vi "Host.vi"() -> ()   [LabVIEW 2018]
uses:
  <instrlib>/niDCPower/nidcpower.llb/niDCPower Measurement Type.ctl
  <instrlib>/niScope/Configure/Trigger/niScope Configure Trigger Window.vi
  <instrlib>/niScope/Acquire/Fetch/niScope Multi Fetch Cluster.vi
  <instrlib>/niScope/Acquire/Fetch/niScope Fetch.vi
panel:
  in  "Tab Control":enum32{"Приборная панель", "Отладочная панель"}(tab)
  in  "STOP":bool=TRUE
  in  "Trigger Source":string(combo)="0"
  in  "AC/DC/Groun":i32(ring)=1 items=["AC", "DC", "Ground"]
  in  "Channel for SEU":T1(radio)
  in  "NI Scope":refnum<k15>="PXI1Slot5_2" caption="Scope"
  in  "High Level":dbl=0.2 format="%.2f"
  in  "Low Level":dbl=-0.2 format="%.2f"
  out "SEU_warning":bool caption="Find SEL"
  out "SEU_Counter":u32 caption="SEU counter"
  out "SEU Waveform":T2(graph) caption="SHUTDOWN Waveform"
  out "RealTime Waveform":T2(graph)=[{"relativeInitialX"=-0.00019999652392947102, "xIncrement"=4e-09, "wfm"=array[100000 elements]}] caption="PC_MON Waveform"
  out "P2 CH1_warning":bool caption="VCC_warning"
  out "P2 CH1_counter":u32 caption="VCC_counter"
  in  "P2 CH1_selcur, A":dbl=0.05 caption="current limit" format="%_6p"
  in  "P2 CH1 Used":bool
  in  "P2 CH1":bool
  out "P2 CH1_char":dbl(graph)=4.1881856349625015e-07
  in  "P2 CH1, V":dbl caption="voltage level" format="%_6p"
  out "P2 CH1_cur, A":dbl=4.1881856349625015e-07 caption="measurement" format="%_6g"
  in  "P2 CH1_curlim, A":dbl=0.1 caption="current limit" format="%_6p"
  out "SEL":bool
  in  "P1 CH0_selcur, A":dbl=0.05 caption="current limit" format="%_6p"
  in  "P1 CH1_selcur, A":dbl=0.05 caption="current limit" format="%_6p"
  in  "P2 CH0_selcur, A":dbl=0.05 caption="current limit" format="%_6p"
  out "P2 CH0_counter":u32 caption="VCC_counter"
  out "P2 CH0_warning":bool caption="VCC_warning"
  out "P1 CH1_counter":u32 caption="VCC_counter"
  out "P1 CH1_warning":bool caption="VCC_warning"
  out "P1 CH0_counter":u32 caption="VCC_counter"
  out "P1 CH0_warning":bool caption="VCC_warning"
  in  "SIM_SEL":bool
  in  "P2 CH0":bool
  in  "P1 CH1":bool
  in  "P1 CH0":bool
  in  "P2 CH0_curlim, A":dbl=0.1 caption="current limit" format="%_6p"
  out "P2 CH0_cur, A":dbl=8.408429577071082e-05 caption="measurement" format="%_6g"
  in  "P2 CH0, V":dbl caption="voltage level" format="%_6p"
  out "P2 CH0_char":dbl(graph)=8.408429577071082e-05
  in  "P1 CH1_curlim, A":dbl=0.1 caption="current limit" format="%_6p"
  out "P1CH1_cur, A":dbl=6.336785656464814e-07 caption="measurement" format="%_6g"
  in  "P1 CH1, V":dbl caption="voltage level" format="%_6p"
  out "P1 CH1_char":dbl(graph)=6.336785656464814e-07
  in  "P1 CH0_curlim, A":dbl=0.1 caption="current limit" format="%_6p"
  out "P1 CH0_cur, A":dbl=0.00010743246200593353 caption="measurement" format="%_6g"
  in  "P1 CH0, V":dbl caption="voltage level" format="%_6p"
  out "P1 CH0_char":dbl(graph)=8.030591065176734e-05
  out "Образец №":string
  in  "POWER 2 (CH0, CH1)":refnum<k15>="PXI1Slot3" caption="PRBS"
  in  "POWER 1 (CH0, CH1)":refnum<k15>="PXI1Slot2" caption="VСС_+5"
  in  "SEU":path=path "D:/NI LabVIEW/8939_VIL/SEU"
  in  "SEL":path=path "D:/NI LabVIEW/8939_VIL/SEL"
  in  "P1 CH0 Used":bool
  in  "P2 CH0 Used":bool
  in  "P1 CH1 Used":bool
  out "SEU last level":dbl
  out "SEU":bool caption="SEL"
  in  "SEL Time Cycle":u32=1
  out "Power OFF":bool
  in  "Считать SIM_SEL":bool
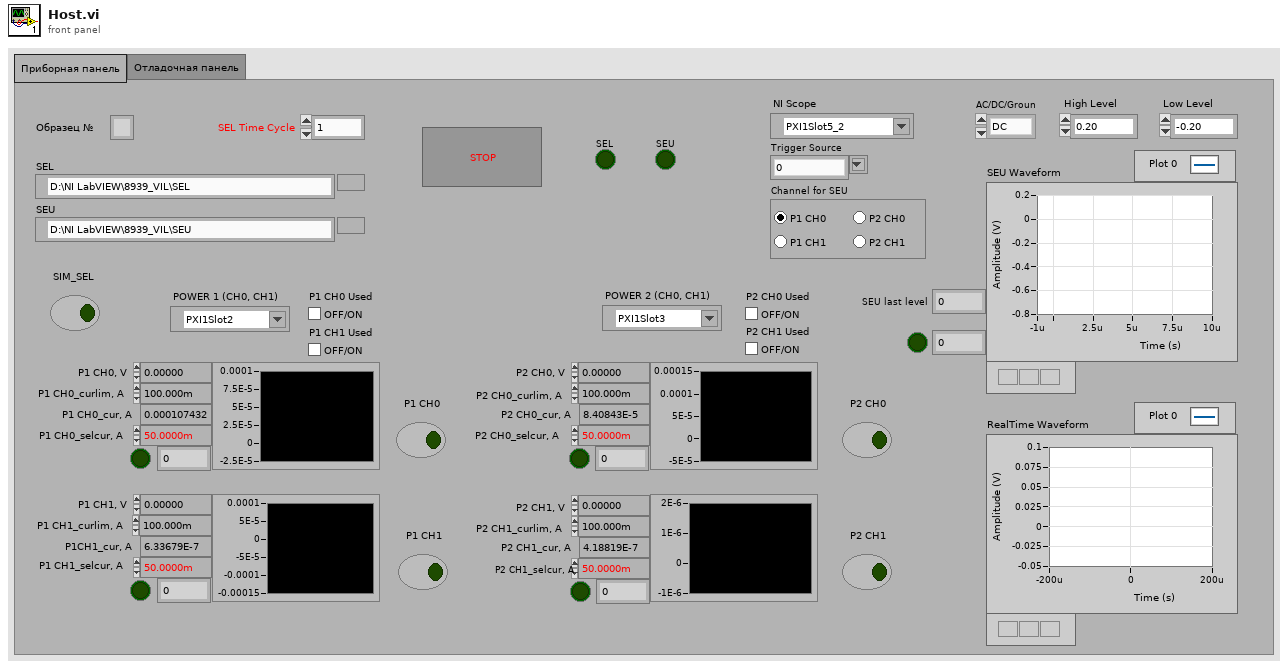
[diagram p1: front panel]
types:
  T1 = enum32{"Radio Selection P1 CH0", "Radio Selection P1 CH1", "Radio Selection P2 CH0", "Radio Selection P2 CH1"}
  T2 = cluster{"relativeInitialX":dbl, "xIncrement":dbl, "wfm":dbl[]}[]
  T3 = enum8{"Enabled", "Disabled", "Disabled and Grayed Out"}
  T4 = enum16{"open", "replace", "create", "open or create", "replace or create", "replace or create with confirmation"}
  T5 = typedef "niDCPower Measurement Type.ctl" = i32
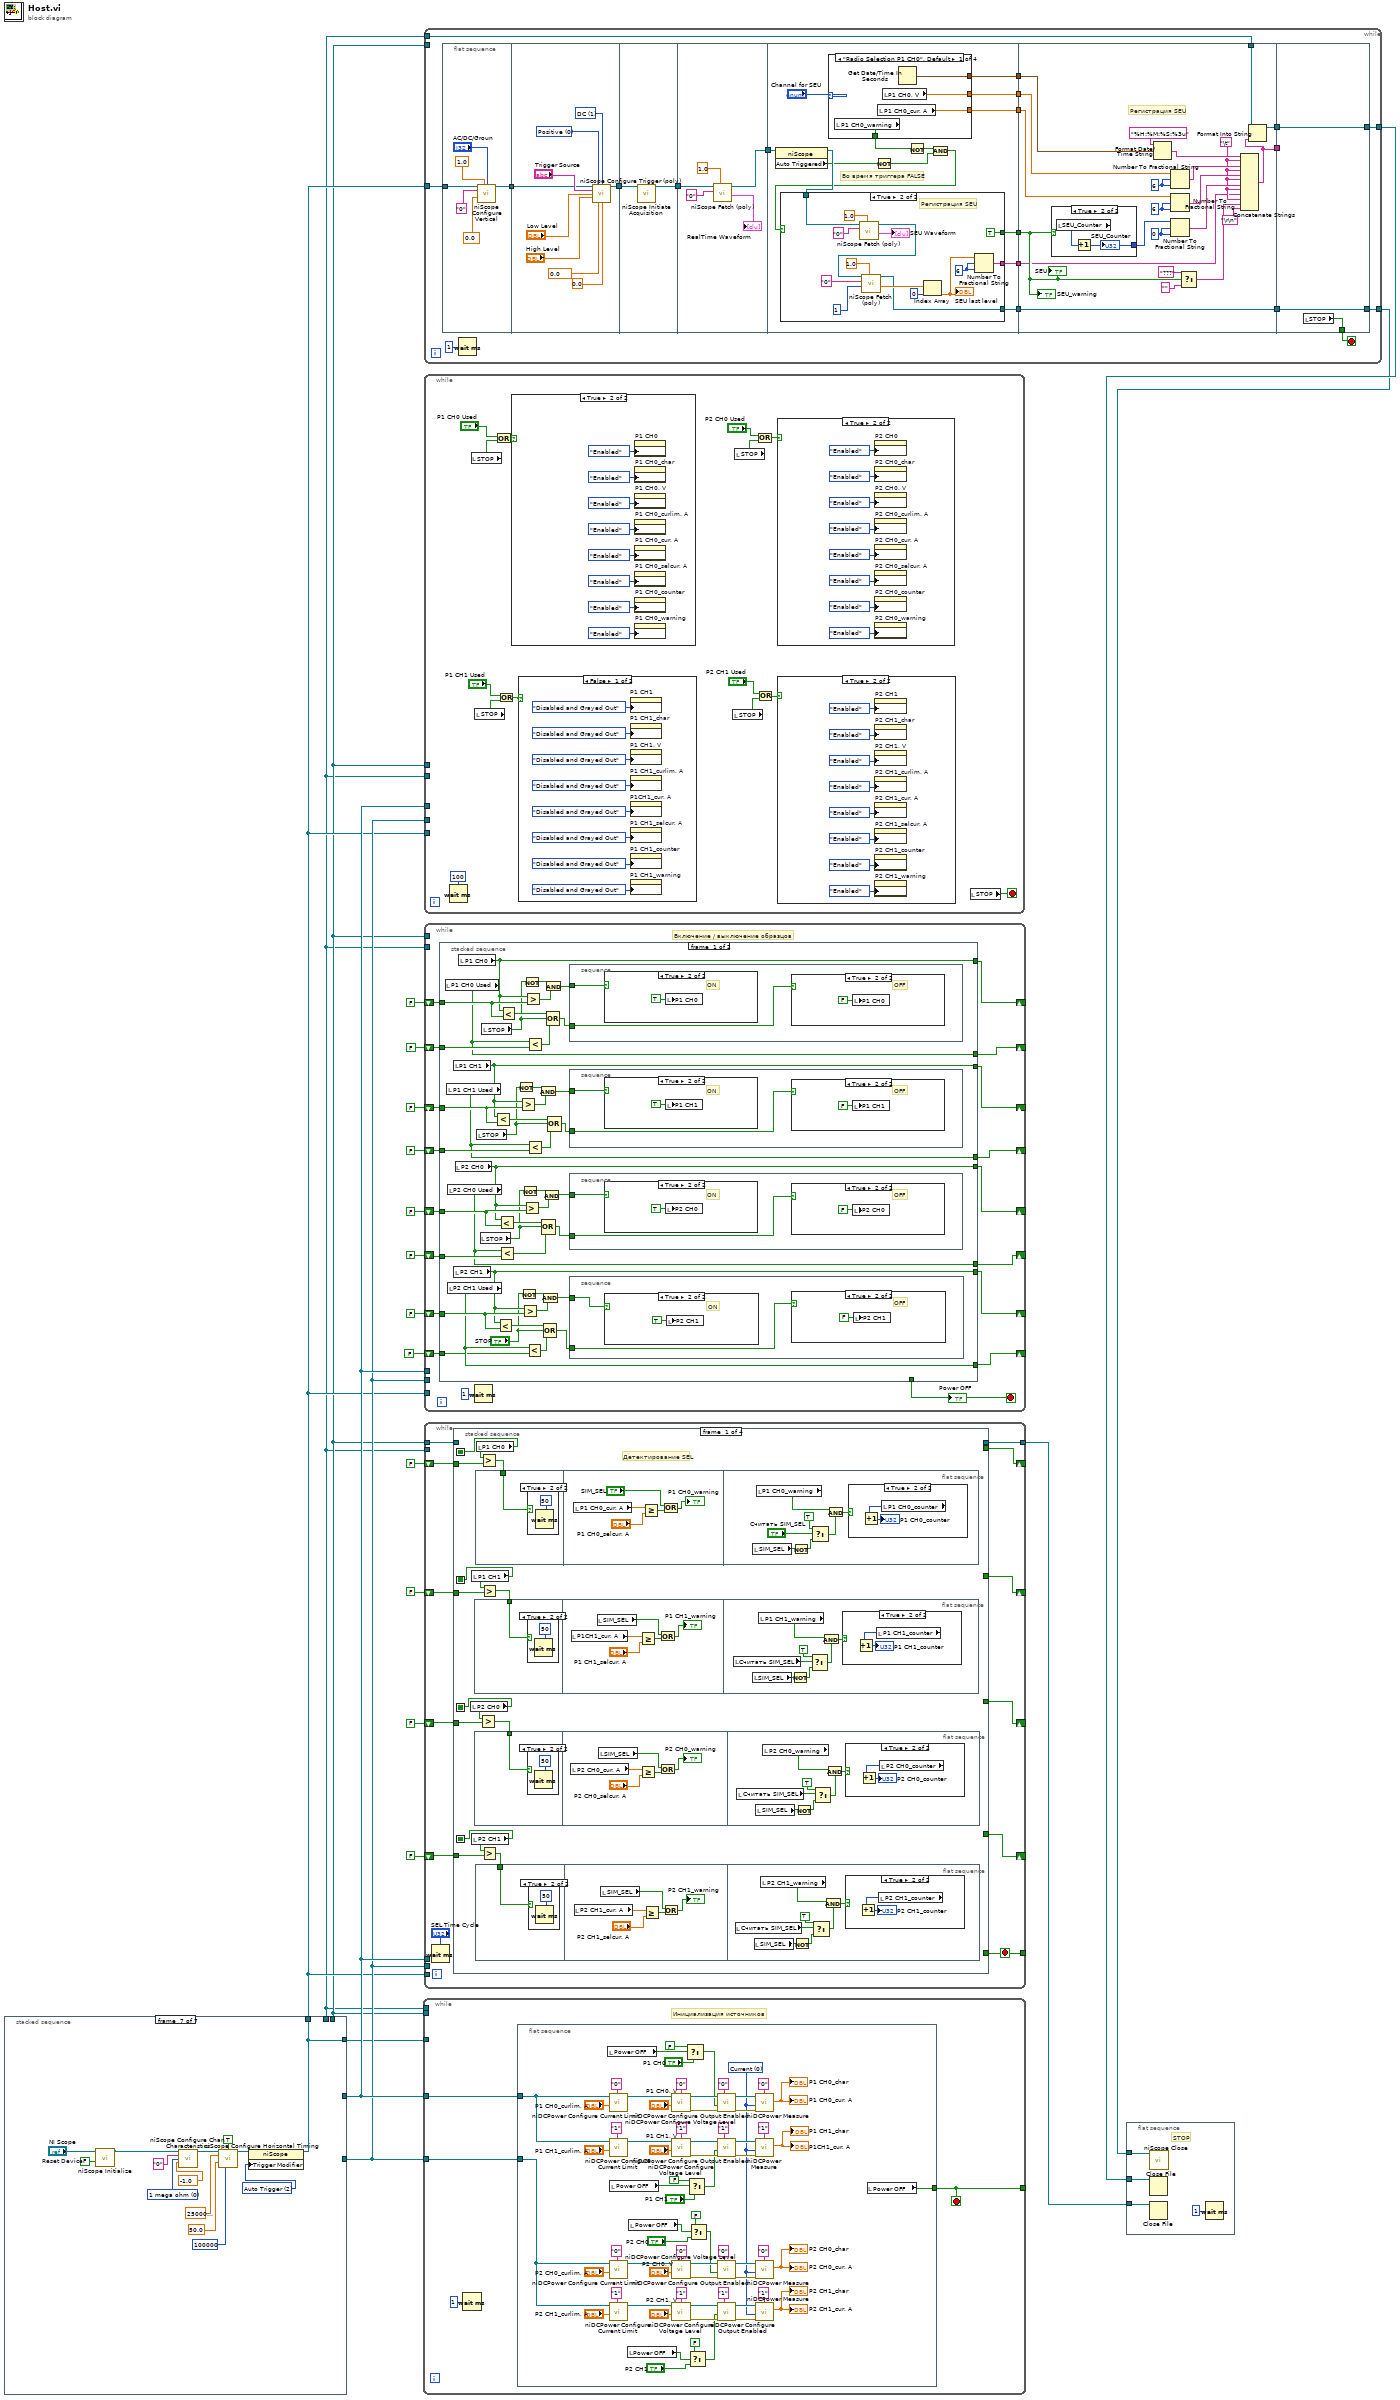
[diagram p0: block diagram]
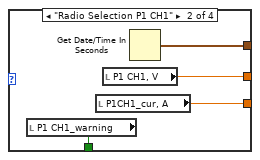
[diagram p2: hidden frame]
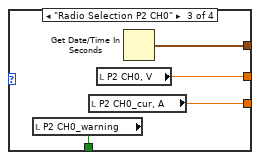
[diagram p3: hidden frame]
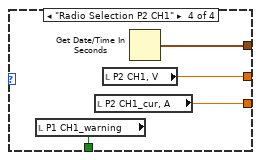
[diagram p4: hidden frame]
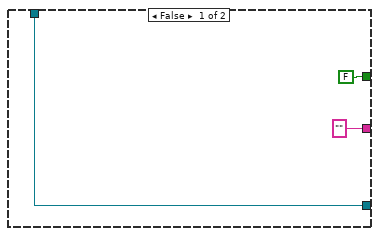
[diagram p5: hidden frame]
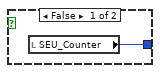
[diagram p6: hidden frame]
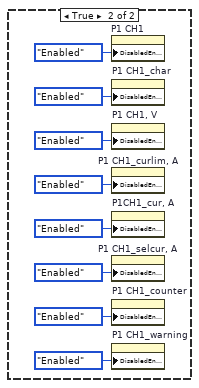
[diagram p7: hidden frame]
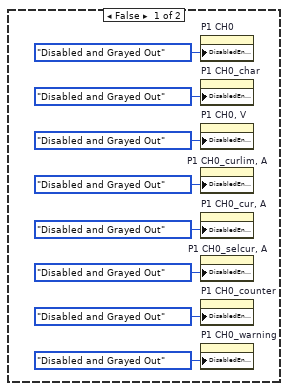
[diagram p8: hidden frame]
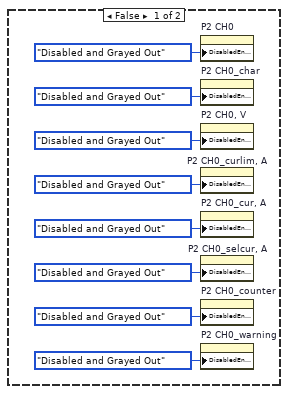
[diagram p9: hidden frame]
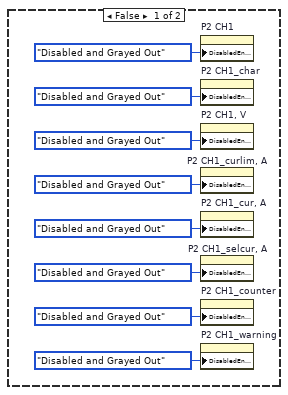
[diagram p10: hidden frame]
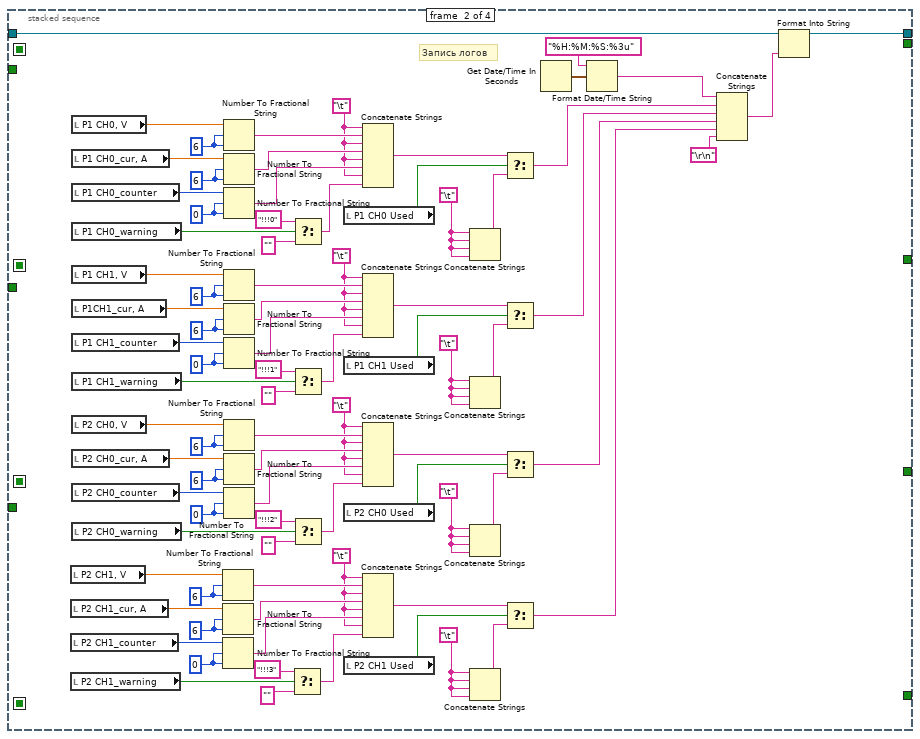
[diagram p19: hidden frame]
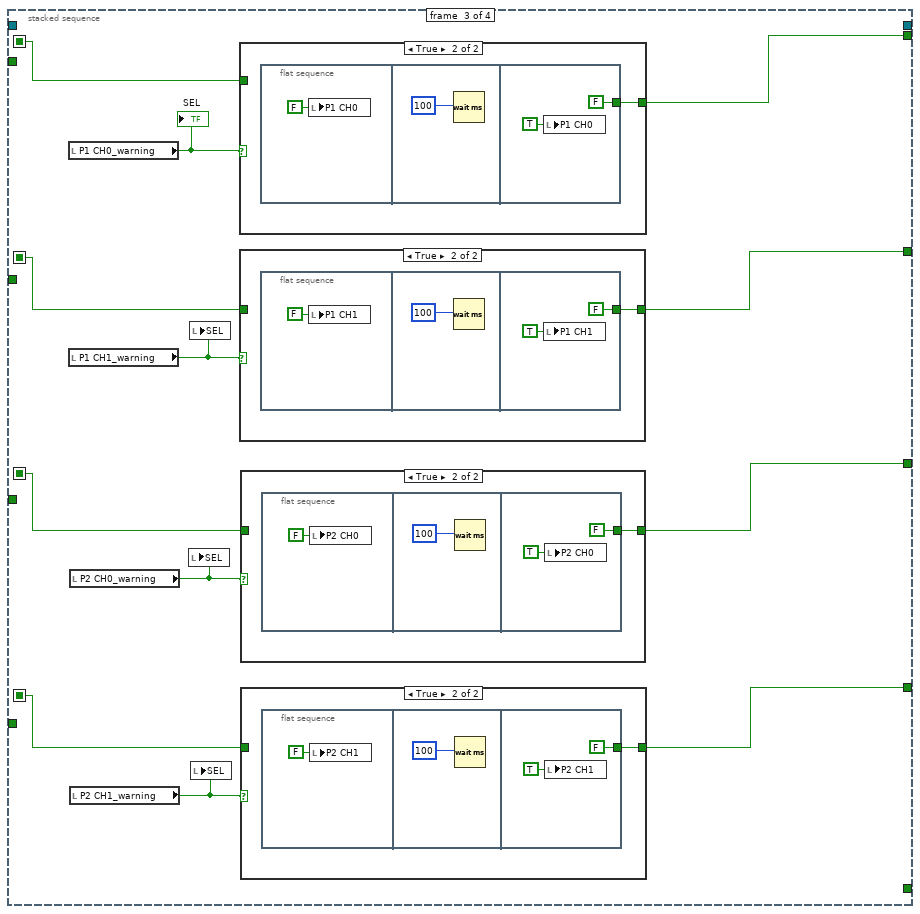
[diagram p20: hidden frame]
diagram:
  n1 = stacked-sequence {
    tunnel: [_ _ _ _ _ w164 _] -> w19
    tunnel: [_ _ _ _ _ w163 _] -> w18
    tunnel: [_ _ _ w97 _ _ _] -> w6
    tunnel: [_ _ _ _ _ _ w175] -> w11
    tunnel: [_ _ _ _ w138 _ _] -> w5
    tunnel: [_ _ _ _ _ _ w175] -> w10
    frame #0 {
      w23 = u32 0 ("SEU_Counter")
      w24 = FALSE ("STOP")
      # "Начальная конфигурация переменных"
      n2 = local write "STOP"(w24) -> ()
      n3 = local write "P1 CH0"(w24) -> ()
      n4 = local write "P1 CH1"(w24) -> ()
      n5 = local write "P2 CH0"(w24) -> ()
      n6 = local write "P2 CH1"(w24) -> ()
      n7 = local write "Power OFF"(w24) -> ()
      n8 = local write "P1 CH0 Used"(w24) -> ()
      n9 = local write "P1 CH1 Used"(w24) -> ()
      n10 = local write "P2 CH0 Used"(w24) -> ()
      n11 = local write "P2 CH1 Used"(w24) -> ()
      n12 = local write "Считать SIM_SEL"(w24) -> ()
      n13 = local write "SEL"(w24) -> ()
      n14 = local write "SEU"(w24) -> ()
      n15 = local write "SEU_warning"(w24) -> ()
      n16 = local write "P1 CH0_warning"(w24) -> ()
      n17 = local write "P1 CH1_warning"(w24) -> ()
      n18 = local write "P2 CH0_warning"(w24) -> ()
      n19 = local write "P2 CH1_warning"(w24) -> ()
      n20 = local write "SEU_warning"(w24) -> ()
      n21 = local write "SEU last level"(0.0 ("SEU Level")) -> ()
      n22 = local write "SEU_Counter"(w23) -> ()
      n23 = local write "P1 CH0_counter"(w23) -> ()
      n24 = local write "P1 CH1_counter"(w23) -> ()
      n25 = local write "P2 CH0_counter"(w23) -> ()
      n26 = local write "P2 CH1_counter"(w23) -> ()
      n27 = local write "Образец №"("" ("Образец №")) -> ()
    }
    frame #1 {
      n28 = stacked-sequence {
        frame #0 {
          n29 = local read "P1 CH0 Used"() -> (w26:bool)
          n30 = case shown="False" w26 {
            frame False {
              n31 = property on="P1 CH0" class="Bool (strict)"("DisabledEnum"=T3."Disabled and Grayed Out" ("Disabled")) -> ()  [unwired: 2 in, 2 out]
              n32 = property on="P1 CH0_char" class="WFChart (strict)"("DisabledEnum"=T3."Disabled and Grayed Out" ("Disabled")) -> ()  [unwired: 2 in, 2 out]
              n33 = property on="P1 CH0, V" class="DigNum (strict)"("DisabledEnum"=T3."Disabled and Grayed Out" ("Disabled")) -> ()  [unwired: 2 in, 2 out]
              n34 = property on="P1 CH0_curlim, A" class="DigNum (strict)"("DisabledEnum"=T3."Disabled and Grayed Out" ("Disabled")) -> ()  [unwired: 2 in, 2 out]
              n35 = property on="P1 CH0_cur, A" class="DigNum (strict)"("DisabledEnum"=T3."Disabled and Grayed Out" ("Disabled")) -> ()  [unwired: 2 in, 2 out]
              n36 = property on="P1 CH0_selcur, A" class="DigNum (strict)"("DisabledEnum"=T3."Disabled and Grayed Out" ("Disabled")) -> ()  [unwired: 2 in, 2 out]
              n37 = property on="P1 CH0_counter" class="DigNum (strict)"("DisabledEnum"=T3."Disabled and Grayed Out" ("Disabled")) -> ()  [unwired: 2 in, 2 out]
              n38 = property on="P1 CH0_warning" class="Bool (strict)"("DisabledEnum"=T3."Disabled and Grayed Out" ("Disabled")) -> ()  [unwired: 2 in, 2 out]
            }
            frame True {
              n39 = property on="P1 CH0" class="Bool (strict)"("DisabledEnum"=T3."Enabled" ("Disabled")) -> ()  [unwired: 2 in, 2 out]
              n40 = property on="P1 CH0_char" class="WFChart (strict)"("DisabledEnum"=T3."Enabled" ("Disabled")) -> ()  [unwired: 2 in, 2 out]
              n41 = property on="P1 CH0, V" class="DigNum (strict)"("DisabledEnum"=T3."Enabled" ("Disabled")) -> ()  [unwired: 2 in, 2 out]
              n42 = property on="P1 CH0_curlim, A" class="DigNum (strict)"("DisabledEnum"=T3."Enabled" ("Disabled")) -> ()  [unwired: 2 in, 2 out]
              n43 = property on="P1 CH0_cur, A" class="DigNum (strict)"("DisabledEnum"=T3."Enabled" ("Disabled")) -> ()  [unwired: 2 in, 2 out]
              n44 = property on="P1 CH0_selcur, A" class="DigNum (strict)"("DisabledEnum"=T3."Enabled" ("Disabled")) -> ()  [unwired: 2 in, 2 out]
              n45 = property on="P1 CH0_counter" class="DigNum (strict)"("DisabledEnum"=T3."Enabled" ("Disabled")) -> ()  [unwired: 2 in, 2 out]
              n46 = property on="P1 CH0_warning" class="Bool (strict)"("DisabledEnum"=T3."Enabled" ("Disabled")) -> ()  [unwired: 2 in, 2 out]
            }
          }
        }
        frame #1 {
          n47 = local read "P1 CH1 Used"() -> (w43:bool)
          n48 = case shown="False" w43 {
            frame False {
              n49 = property on="P1 CH1" class="Bool (strict)"("DisabledEnum"=T3."Disabled and Grayed Out" ("Disabled")) -> ()  [unwired: 2 in, 2 out]
              n50 = property on="P1 CH1_char" class="WFChart (strict)"("DisabledEnum"=T3."Disabled and Grayed Out" ("Disabled")) -> ()  [unwired: 2 in, 2 out]
              n51 = property on="P1 CH1, V" class="DigNum (strict)"("DisabledEnum"=T3."Disabled and Grayed Out" ("Disabled")) -> ()  [unwired: 2 in, 2 out]
              n52 = property on="P1 CH1_curlim, A" class="DigNum (strict)"("DisabledEnum"=T3."Disabled and Grayed Out" ("Disabled")) -> ()  [unwired: 2 in, 2 out]
              n53 = property on="P1CH1_cur, A" class="DigNum (strict)"("DisabledEnum"=T3."Disabled and Grayed Out" ("Disabled")) -> ()  [unwired: 2 in, 2 out]
              n54 = property on="P1 CH1_selcur, A" class="DigNum (strict)"("DisabledEnum"=T3."Disabled and Grayed Out" ("Disabled")) -> ()  [unwired: 2 in, 2 out]
              n55 = property on="P1 CH1_counter" class="DigNum (strict)"("DisabledEnum"=T3."Disabled and Grayed Out" ("Disabled")) -> ()  [unwired: 2 in, 2 out]
              n56 = property on="P1 CH1_warning" class="Bool (strict)"("DisabledEnum"=T3."Disabled and Grayed Out" ("Disabled")) -> ()  [unwired: 2 in, 2 out]
            }
            frame True {
              n57 = property on="P1 CH1" class="Bool (strict)"("DisabledEnum"=T3."Enabled" ("Disabled")) -> ()  [unwired: 2 in, 2 out]
              n58 = property on="P1 CH1_char" class="WFChart (strict)"("DisabledEnum"=T3."Enabled" ("Disabled")) -> ()  [unwired: 2 in, 2 out]
              n59 = property on="P1 CH1, V" class="DigNum (strict)"("DisabledEnum"=T3."Enabled" ("Disabled")) -> ()  [unwired: 2 in, 2 out]
              n60 = property on="P1 CH1_curlim, A" class="DigNum (strict)"("DisabledEnum"=T3."Enabled" ("Disabled")) -> ()  [unwired: 2 in, 2 out]
              n61 = property on="P1CH1_cur, A" class="DigNum (strict)"("DisabledEnum"=T3."Enabled" ("Disabled")) -> ()  [unwired: 2 in, 2 out]
              n62 = property on="P1 CH1_selcur, A" class="DigNum (strict)"("DisabledEnum"=T3."Enabled" ("Disabled")) -> ()  [unwired: 2 in, 2 out]
              n63 = property on="P1 CH1_counter" class="DigNum (strict)"("DisabledEnum"=T3."Enabled" ("Disabled")) -> ()  [unwired: 2 in, 2 out]
              n64 = property on="P1 CH1_warning" class="Bool (strict)"("DisabledEnum"=T3."Enabled" ("Disabled")) -> ()  [unwired: 2 in, 2 out]
            }
          }
        }
        frame #2 {
          n65 = local read "P2 CH0 Used"() -> (w60:bool)
          n66 = case shown="False" w60 {
            frame False {
              n67 = property on="P2 CH0" class="Bool (strict)"("DisabledEnum"=T3."Disabled and Grayed Out" ("Disabled")) -> ()  [unwired: 2 in, 2 out]
              n68 = property on="P2 CH0_char" class="WFChart (strict)"("DisabledEnum"=T3."Disabled and Grayed Out" ("Disabled")) -> ()  [unwired: 2 in, 2 out]
              n69 = property on="P2 CH0, V" class="DigNum (strict)"("DisabledEnum"=T3."Disabled and Grayed Out" ("Disabled")) -> ()  [unwired: 2 in, 2 out]
              n70 = property on="P2 CH0_curlim, A" class="DigNum (strict)"("DisabledEnum"=T3."Disabled and Grayed Out" ("Disabled")) -> ()  [unwired: 2 in, 2 out]
              n71 = property on="P2 CH0_cur, A" class="DigNum (strict)"("DisabledEnum"=T3."Disabled and Grayed Out" ("Disabled")) -> ()  [unwired: 2 in, 2 out]
              n72 = property on="P2 CH0_selcur, A" class="DigNum (strict)"("DisabledEnum"=T3."Disabled and Grayed Out" ("Disabled")) -> ()  [unwired: 2 in, 2 out]
              n73 = property on="P2 CH0_counter" class="DigNum (strict)"("DisabledEnum"=T3."Disabled and Grayed Out" ("Disabled")) -> ()  [unwired: 2 in, 2 out]
              n74 = property on="P2 CH0_warning" class="Bool (strict)"("DisabledEnum"=T3."Disabled and Grayed Out" ("Disabled")) -> ()  [unwired: 2 in, 2 out]
            }
            frame True {
              n75 = property on="P2 CH0" class="Bool (strict)"("DisabledEnum"=T3."Enabled" ("Disabled")) -> ()  [unwired: 2 in, 2 out]
              n76 = property on="P2 CH0_char" class="WFChart (strict)"("DisabledEnum"=T3."Enabled" ("Disabled")) -> ()  [unwired: 2 in, 2 out]
              n77 = property on="P2 CH0, V" class="DigNum (strict)"("DisabledEnum"=T3."Enabled" ("Disabled")) -> ()  [unwired: 2 in, 2 out]
              n78 = property on="P2 CH0_curlim, A" class="DigNum (strict)"("DisabledEnum"=T3."Enabled" ("Disabled")) -> ()  [unwired: 2 in, 2 out]
              n79 = property on="P2 CH0_cur, A" class="DigNum (strict)"("DisabledEnum"=T3."Enabled" ("Disabled")) -> ()  [unwired: 2 in, 2 out]
              n80 = property on="P2 CH0_selcur, A" class="DigNum (strict)"("DisabledEnum"=T3."Enabled" ("Disabled")) -> ()  [unwired: 2 in, 2 out]
              n81 = property on="P2 CH0_counter" class="DigNum (strict)"("DisabledEnum"=T3."Enabled" ("Disabled")) -> ()  [unwired: 2 in, 2 out]
              n82 = property on="P2 CH0_warning" class="Bool (strict)"("DisabledEnum"=T3."Enabled" ("Disabled")) -> ()  [unwired: 2 in, 2 out]
            }
          }
        }
        frame #3 {
          n83 = local read "P2 CH1 Used"() -> (w77:bool)
          n84 = case shown="True" w77 {
            frame False {
              n85 = property on="P2 CH1" class="Bool (strict)"("DisabledEnum"=T3."Disabled and Grayed Out" ("Disabled")) -> ()  [unwired: 2 in, 2 out]
              n86 = property on="P2 CH1_char" class="WFChart (strict)"("DisabledEnum"=T3."Disabled and Grayed Out" ("Disabled")) -> ()  [unwired: 2 in, 2 out]
              n87 = property on="P2 CH1, V" class="DigNum (strict)"("DisabledEnum"=T3."Disabled and Grayed Out" ("Disabled")) -> ()  [unwired: 2 in, 2 out]
              n88 = property on="P2 CH1_curlim, A" class="DigNum (strict)"("DisabledEnum"=T3."Disabled and Grayed Out" ("Disabled")) -> ()  [unwired: 2 in, 2 out]
              n89 = property on="P2 CH1_cur, A" class="DigNum (strict)"("DisabledEnum"=T3."Disabled and Grayed Out" ("Disabled")) -> ()  [unwired: 2 in, 2 out]
              n90 = property on="P2 CH1_selcur, A" class="DigNum (strict)"("DisabledEnum"=T3."Disabled and Grayed Out" ("Disabled")) -> ()  [unwired: 2 in, 2 out]
              n91 = property on="P2 CH1_counter" class="DigNum (strict)"("DisabledEnum"=T3."Disabled and Grayed Out" ("Disabled")) -> ()  [unwired: 2 in, 2 out]
              n92 = property on="P2 CH1_warning" class="Bool (strict)"("DisabledEnum"=T3."Disabled and Grayed Out" ("Disabled")) -> ()  [unwired: 2 in, 2 out]
            }
            frame True {
              n93 = property on="P2 CH1" class="Bool (strict)"("DisabledEnum"=T3."Enabled" ("Disabled")) -> ()  [unwired: 2 in, 2 out]
              n94 = property on="P2 CH1_char" class="WFChart (strict)"("DisabledEnum"=T3."Enabled" ("Disabled")) -> ()  [unwired: 2 in, 2 out]
              n95 = property on="P2 CH1, V" class="DigNum (strict)"("DisabledEnum"=T3."Enabled" ("Disabled")) -> ()  [unwired: 2 in, 2 out]
              n96 = property on="P2 CH1_curlim, A" class="DigNum (strict)"("DisabledEnum"=T3."Enabled" ("Disabled")) -> ()  [unwired: 2 in, 2 out]
              n97 = property on="P2 CH1_cur, A" class="DigNum (strict)"("DisabledEnum"=T3."Enabled" ("Disabled")) -> ()  [unwired: 2 in, 2 out]
              n98 = property on="P2 CH1_selcur, A" class="DigNum (strict)"("DisabledEnum"=T3."Enabled" ("Disabled")) -> ()  [unwired: 2 in, 2 out]
              n99 = property on="P2 CH1_counter" class="DigNum (strict)"("DisabledEnum"=T3."Enabled" ("Disabled")) -> ()  [unwired: 2 in, 2 out]
              n100 = property on="P2 CH1_warning" class="Bool (strict)"("DisabledEnum"=T3."Enabled" ("Disabled")) -> ()  [unwired: 2 in, 2 out]
            }
          }
        }
      }
    }
    frame #2 {
      n101 = call "Begin.vi"() -> ("Образец № 2"=→"Образец №":string)  [unwired: 9 in]
    }
    frame #3 {
      w96 = "\t"
      # "Инициализация файла SEL"
      n102 = local read "Образец №"() -> (w116:string)
      n103 = Build Path(base path="SEL", name or relative path=w116) -> (appended path=w131:path)
      n104 = Get Date/Time In Seconds() -> (seconds since 1Jan1904=w127:timestamp)
      n105 = call <vilib>:"Check if File or Folder Exists.vi"("path"=w131) -> ("file or folder exists?"=w130:bool, "dup path"=w129:path)  [unwired: 8 in, 1 out]
      n106 = Format Date/Time String(time format string (%c)="SEL %d %m %y %H.%M.%S", seconds (now)=w127) -> (date/time string=w126:string)  [unwired: 1 in]
      n107 = case shown="False" w130 {
        tunnel: w129 -> [w133 w134]
        tunnel: [w132 w134] -> w128
        frame False {
          n108 = Create Folder(path (use dialog)=w133) -> (created path=w132:path)  [unwired: 2 in, 2 out]
        }
        frame True {
        }
      }
      n109 = Concatenate Strings(w126, ".xls" ("string")) -> (w123:string)
      n110 = Build Path(base path=w128, name or relative path=w123) -> (appended path=w120:path)
      n111 = Open/Create/Replace File(file path (use dialog)=w120, operation (0:open)=T4."open or create", access (0:read/write)=enum16{"read/write", "read-only", "write-only"}."read/write") -> (refnum out=w119:refnum<file>)  [unwired: 3 in, 2 out]
      n112 = Set File Position(refnum=w119, from (0:start)=enum16{"start", "end", "current"}."end") -> (refnum out=w98:refnum<file>)  [unwired: 2 in, 1 out]
      n113 = Format Into String(initial string=w98, "Time" ("string"), w96, "P1 CH0, V" ("string"), w96, "P1 CH0_cur, A" ("string"), w96, "P1 CH0_counter" ("string"), w96, "!!!0" ("input 7"), w96, "P1 CH1, V" ("string"), w96, "P1 CH1_cur, A" ("string"), w96, "P1 CH1_counter" ("string"), w96, "!!!1" ("input 7"), w96, "P2 CH0, V" ("string"), w96, "P2 CH0_cur, A" ("string"), w96, "P2 CH0_counter" ("string"), w96, "!!!2" ("input 7"), w96, "P2 CH1, V" ("string"), w96, "P2 CH1_cur, A" ("string"), w96, "P2 CH1_counter" ("string"), "!!!3" ("input 7"), "\r\n") -> (resulting string=w97:refnum<file>)  [unwired: 2 in, 1 out]
    }
    frame #4 {
      w137 = "\t"
      # "Инициализация файла SEU"
      n114 = local read "Образец №"() -> (w149:string)
      n115 = Build Path(base path="SEU", name or relative path=w149) -> (appended path=w159:path)
      n116 = Get Date/Time In Seconds() -> (seconds since 1Jan1904=w155:timestamp)
      n117 = call <vilib>:"Check if File or Folder Exists.vi"("path"=w159) -> ("file or folder exists?"=w158:bool, "dup path"=w157:path)  [unwired: 8 in, 1 out]
      n118 = Format Date/Time String(time format string (%c)="SEU %d %m %y %H.%M.%S", seconds (now)=w155) -> (date/time string=w154:string)  [unwired: 1 in]
      n119 = case shown="False" w158 {
        tunnel: w157 -> [w161 w162]
        tunnel: [w160 w162] -> w156
        frame False {
          n120 = Create Folder(path (use dialog)=w161) -> (created path=w160:path)  [unwired: 2 in, 2 out]
        }
        frame True {
        }
      }
      n121 = Concatenate Strings(w154, ".xls" ("string")) -> (w153:string)
      n122 = Build Path(base path=w156, name or relative path=w153) -> (appended path=w152:path)
      n123 = Open/Create/Replace File(file path (use dialog)=w152, operation (0:open)=T4."open or create", access (0:read/write)=enum16{"read/write", "read-only", "write-only"}."read/write") -> (refnum out=w151:refnum<file>)  [unwired: 3 in, 2 out]
      n124 = Set File Position(refnum=w151, from (0:start)=enum16{"start", "end", "current"}."end") -> (refnum out=w139:refnum<file>)  [unwired: 2 in, 1 out]
      n125 = Format Into String(initial string=w139, "Time" ("string"), w137, "Voltage, V" ("string"), w137, "Current, A" ("string"), w137, "SEU counter" ("string"), w137, "!!!" ("input 7"), "\r\n") -> (resulting string=w138:refnum<file>)  [unwired: 2 in, 1 out]
    }
    frame #5 {
      # "Инициализация источника"
      n126 = call <instrlib>:"niDCPower Initialize.vi"("resource name"="POWER 1 (CH0, CH1)") -> ("error out"=w173:errorcluster, "instrument handle out"=w174:refnum<k15>)  [unwired: 3 in, 6 out]
      n127 = call <instrlib>:"niDCPower Initialize.vi"("resource name"="POWER 2 (CH0, CH1)") -> ("error out"=w170:errorcluster, "instrument handle out"=w171:refnum<k15>)  [unwired: 3 in, 6 out]
      n128 = call <instrlib>:"niDCPower Configure Voltage Level.vi"("error in (no error)"=w173, "voltage level"=0.0, "channel name"="0,1", "instrument handle"=w174) -> ("instrument handle out"=w164:refnum<k15>)  [unwired: 6 in, 1 out]
      n129 = call <instrlib>:"niDCPower Configure Voltage Level.vi"("error in (no error)"=w170, "voltage level"=0.0, "channel name"="0,1", "instrument handle"=w171) -> ("instrument handle out"=w163:refnum<k15>)  [unwired: 6 in, 1 out]
    }
    frame #6 {
      w179 = 2 items=["None"=1, "Auto Trigger"=2] ("Triggering:Trigger Modifier")
      w185 = u32 0 items=["1 mega ohm"=0, "50 ohms"=2] ("Input Impedance")
      w187 = FALSE  # Reset Device
      n130 = call <instrlib>:"niScope Initialize.vi"("resource name"="NI Scope", "reset device"=w187) -> ("instrument handle"=w176:refnum<k15>)  [unwired: 12 in, 1 out]
      n131 = call <instrlib>:"niScope Configure Chan Characteristics.vi"("instrument handle"=w176, "channels"="0" ("Channel Name"), "input impedance"=w185, "maximum input frequency"=-1.0 ("Maximum Input Frequency")) -> ("instrument handle out"=w178:refnum<k15>)  [unwired: 10 in, 1 out]
      n132 = call <instrlib>:"niScope Configure Horizontal Timing.vi"("instrument handle"=w178, "enforce realtime"=TRUE ("Enforce Realtime"), "min sample rate"=250000000.0 ("Min Sample Rate"), "reference position"=50.0 ("Reference\nPosition"), "min record length"=100000 ("Min Record Length")) -> ("instrument handle out"=w177:refnum<k15>)  [unwired: 9 in, 1 out]
      n133 = property on="Property Node" class="niScope"(reference=w177, "Trigger Modifier"=w179) -> (reference out=w175:refnum<k15>)  [unwired: 1 in, 1 out]
    }
  }
  n134 = while {
    tunnel: w19 -> [w192]
    tunnel: [w191] -> _
    tunnel: w18 -> [w189]
    tunnel: w10 -> [_]
    tunnel: w6 -> [_]
    tunnel: w5 -> [_]
    stop <- w191 stop-if-true
    # "Инициализация источников"
    n135 = Wait (ms)(milliseconds to wait=u32 1) -> ()  [unwired: 1 out]
    n136 = flat-sequence {
      tunnel: w192 -> [w260]
      tunnel: [w235] -> w191
      tunnel: w189 -> [w193]
      frame #0 {
        w194 = T5 0 items=["Current", "Voltage"] ("measurement type")
        n137 = local read "Power OFF"() -> (w212:bool)
        n138 = call <instrlib>:"niDCPower Configure Current Limit.vi"("current limit"="P1 CH0_curlim, A", "channel name"="0", "instrument handle"=w260) -> ("instrument handle out"=w249:refnum<k15>)  [unwired: 7 in, 1 out]
        n139 = call <instrlib>:"niDCPower Configure Current Limit.vi"("current limit"="P1 CH1_curlim, A", "channel name"="1", "instrument handle"=w260) -> ("instrument handle out"=w246:refnum<k15>)  [unwired: 7 in, 1 out]
        n140 = call <instrlib>:"niDCPower Configure Current Limit.vi"("current limit"="P2 CH0_curlim, A", "channel name"="0", "instrument handle"=w193) -> ("instrument handle out"=w225:refnum<k15>)  [unwired: 7 in, 1 out]
        n141 = call <instrlib>:"niDCPower Configure Current Limit.vi"("current limit"="P2 CH1_curlim, A", "channel name"="1", "instrument handle"=w193) -> ("instrument handle out"=w204:refnum<k15>)  [unwired: 7 in, 1 out]
        n142 = local read "Power OFF"() -> (w234:bool)
        n143 = local read "Power OFF"() -> (w197:bool)
        n144 = local read "Power OFF"() -> (w217:bool)
        n145 = call <instrlib>:"niDCPower Configure Voltage Level.vi"("voltage level"="P1 CH0, V", "channel name"="0", "instrument handle"=w249) -> ("error out"=w254:errorcluster, "instrument handle out"=w255:refnum<k15>)  [unwired: 7 in]
        n146 = call <instrlib>:"niDCPower Configure Voltage Level.vi"("voltage level"="P1 CH1, V", "channel name"="1", "instrument handle"=w246) -> ("error out"=w252:errorcluster, "instrument handle out"=w253:refnum<k15>)  [unwired: 7 in]
        n147 = call <instrlib>:"niDCPower Configure Voltage Level.vi"("voltage level"="P2 CH0, V", "channel name"="0", "instrument handle"=w225) -> ("error out"=w222:errorcluster, "instrument handle out"=w221:refnum<k15>)  [unwired: 7 in]
        n148 = call <instrlib>:"niDCPower Configure Voltage Level.vi"("voltage level"="P2 CH1, V", "channel name"="1", "instrument handle"=w204) -> ("error out"=w207:errorcluster, "instrument handle out"=w208:refnum<k15>)  [unwired: 7 in]
        n149 = Select(t=FALSE, s=w212, f="P1 CH0") -> (s? t:f=w211:bool)
        n150 = Select(t=FALSE, s=w234, f="P1 CH1") -> (s? t:f=w231:bool)
        n151 = Select(t=FALSE, s=w197, f="P2 CH1") -> (s? t:f=w195:bool)
        n152 = Select(t=FALSE, s=w217, f="P2 CH0") -> (s? t:f=w216:bool)
        n153 = call <instrlib>:"niDCPower Configure Output Enabled.vi"("error in (no error)"=w254, "output enabled"=w211, "channel name"="0", "instrument handle"=w255) -> ("error out"=w257:errorcluster, "instrument handle out"=w256:refnum<k15>)  [unwired: 6 in]
        n154 = call <instrlib>:"niDCPower Configure Output Enabled.vi"("error in (no error)"=w252, "output enabled"=w231, "channel name"="1", "instrument handle"=w253) -> ("error out"=w259:errorcluster, "instrument handle out"=w258:refnum<k15>)  [unwired: 6 in]
        n155 = call <instrlib>:"niDCPower Configure Output Enabled.vi"("error in (no error)"=w222, "output enabled"=w216, "channel name"="0", "instrument handle"=w221) -> ("error out"=w219:errorcluster, "instrument handle out"=w220:refnum<k15>)  [unwired: 6 in]
        n156 = call <instrlib>:"niDCPower Configure Output Enabled.vi"("error in (no error)"=w207, "output enabled"=w195, "channel name"="1", "instrument handle"=w208) -> ("error out"=w210:errorcluster, "instrument handle out"=w209:refnum<k15>)  [unwired: 6 in]
        n157 = call <instrlib>:"niDCPower Measure.vi"("error in (no error)"=w257, "measurement type"=w194, "channel name"="0", "instrument handle"=w256) -> ("measurement"=→"P1 CH0_cur, A" →"P1 CH0_char":dbl)  [unwired: 5 in, 2 out]
        n158 = call <instrlib>:"niDCPower Measure.vi"("error in (no error)"=w259, "measurement type"=w194, "channel name"="1", "instrument handle"=w258) -> ("measurement"=→"P1CH1_cur, A" →"P1 CH1_char":dbl)  [unwired: 5 in, 2 out]
        n159 = call <instrlib>:"niDCPower Measure.vi"("error in (no error)"=w219, "measurement type"=w194, "channel name"="0", "instrument handle"=w220) -> ("measurement"=→"P2 CH0_cur, A" →"P2 CH0_char":dbl)  [unwired: 5 in, 2 out]
        n160 = call <instrlib>:"niDCPower Measure.vi"("error in (no error)"=w210, "measurement type"=w194, "channel name"="1", "instrument handle"=w209) -> ("measurement"=→"P2 CH1_cur, A" →"P2 CH1_char":dbl)  [unwired: 5 in, 2 out]
        n161 = local read "Power OFF"() -> (w235:bool)
      }
    }
  }
  n162 = while {
    tunnel: w19 -> [_]
    tunnel: w18 -> [_]
    tunnel: w6 -> [_]
    tunnel: w5 -> [_]
    tunnel: w11 -> [_]
    stop <- w274 stop-if-true
    n163 = Wait (ms)(milliseconds to wait=u32 100) -> ()  [unwired: 1 out]
    n164 = local read "STOP"() -> (w264:bool)
    n165 = local read "STOP"() -> (w261:bool)
    n166 = Or(x="P1 CH0 Used", y=w264) -> (x .or. y?=w266:bool)
    n167 = Or(x="P1 CH1 Used", y=w261) -> (x .or. y?=w263:bool)
    n168 = case shown="True" w266 {
      frame False {
        n169 = property on="P1 CH0" class="Bool (strict)"("DisabledEnum"=T3."Disabled and Grayed Out" ("Disabled")) -> ()  [unwired: 2 in, 2 out]
        n170 = property on="P1 CH0_char" class="WFChart (strict)"("DisabledEnum"=T3."Disabled and Grayed Out" ("Disabled")) -> ()  [unwired: 2 in, 2 out]
        n171 = property on="P1 CH0, V" class="DigNum (strict)"("DisabledEnum"=T3."Disabled and Grayed Out" ("Disabled")) -> ()  [unwired: 2 in, 2 out]
        n172 = property on="P1 CH0_curlim, A" class="DigNum (strict)"("DisabledEnum"=T3."Disabled and Grayed Out" ("Disabled")) -> ()  [unwired: 2 in, 2 out]
        n173 = property on="P1 CH0_cur, A" class="DigNum (strict)"("DisabledEnum"=T3."Disabled and Grayed Out" ("Disabled")) -> ()  [unwired: 2 in, 2 out]
        n174 = property on="P1 CH0_selcur, A" class="DigNum (strict)"("DisabledEnum"=T3."Disabled and Grayed Out" ("Disabled")) -> ()  [unwired: 2 in, 2 out]
        n175 = property on="P1 CH0_counter" class="DigNum (strict)"("DisabledEnum"=T3."Disabled and Grayed Out" ("Disabled")) -> ()  [unwired: 2 in, 2 out]
        n176 = property on="P1 CH0_warning" class="Bool (strict)"("DisabledEnum"=T3."Disabled and Grayed Out" ("Disabled")) -> ()  [unwired: 2 in, 2 out]
      }
      frame True {
        n177 = property on="P1 CH0" class="Bool (strict)"("DisabledEnum"=T3."Enabled" ("Disabled")) -> ()  [unwired: 2 in, 2 out]
        n178 = property on="P1 CH0_char" class="WFChart (strict)"("DisabledEnum"=T3."Enabled" ("Disabled")) -> ()  [unwired: 2 in, 2 out]
        n179 = property on="P1 CH0, V" class="DigNum (strict)"("DisabledEnum"=T3."Enabled" ("Disabled")) -> ()  [unwired: 2 in, 2 out]
        n180 = property on="P1 CH0_curlim, A" class="DigNum (strict)"("DisabledEnum"=T3."Enabled" ("Disabled")) -> ()  [unwired: 2 in, 2 out]
        n181 = property on="P1 CH0_cur, A" class="DigNum (strict)"("DisabledEnum"=T3."Enabled" ("Disabled")) -> ()  [unwired: 2 in, 2 out]
        n182 = property on="P1 CH0_selcur, A" class="DigNum (strict)"("DisabledEnum"=T3."Enabled" ("Disabled")) -> ()  [unwired: 2 in, 2 out]
        n183 = property on="P1 CH0_counter" class="DigNum (strict)"("DisabledEnum"=T3."Enabled" ("Disabled")) -> ()  [unwired: 2 in, 2 out]
        n184 = property on="P1 CH0_warning" class="Bool (strict)"("DisabledEnum"=T3."Enabled" ("Disabled")) -> ()  [unwired: 2 in, 2 out]
      }
    }
    n185 = case shown="False" w263 {
      frame False {
        n186 = property on="P1 CH1" class="Bool (strict)"("DisabledEnum"=T3."Disabled and Grayed Out" ("Disabled")) -> ()  [unwired: 2 in, 2 out]
        n187 = property on="P1 CH1_char" class="WFChart (strict)"("DisabledEnum"=T3."Disabled and Grayed Out" ("Disabled")) -> ()  [unwired: 2 in, 2 out]
        n188 = property on="P1 CH1, V" class="DigNum (strict)"("DisabledEnum"=T3."Disabled and Grayed Out" ("Disabled")) -> ()  [unwired: 2 in, 2 out]
        n189 = property on="P1 CH1_curlim, A" class="DigNum (strict)"("DisabledEnum"=T3."Disabled and Grayed Out" ("Disabled")) -> ()  [unwired: 2 in, 2 out]
        n190 = property on="P1CH1_cur, A" class="DigNum (strict)"("DisabledEnum"=T3."Disabled and Grayed Out" ("Disabled")) -> ()  [unwired: 2 in, 2 out]
        n191 = property on="P1 CH1_selcur, A" class="DigNum (strict)"("DisabledEnum"=T3."Disabled and Grayed Out" ("Disabled")) -> ()  [unwired: 2 in, 2 out]
        n192 = property on="P1 CH1_counter" class="DigNum (strict)"("DisabledEnum"=T3."Disabled and Grayed Out" ("Disabled")) -> ()  [unwired: 2 in, 2 out]
        n193 = property on="P1 CH1_warning" class="Bool (strict)"("DisabledEnum"=T3."Disabled and Grayed Out" ("Disabled")) -> ()  [unwired: 2 in, 2 out]
      }
      frame True {
        n194 = property on="P1 CH1" class="Bool (strict)"("DisabledEnum"=T3."Enabled" ("Disabled")) -> ()  [unwired: 2 in, 2 out]
        n195 = property on="P1 CH1_char" class="WFChart (strict)"("DisabledEnum"=T3."Enabled" ("Disabled")) -> ()  [unwired: 2 in, 2 out]
        n196 = property on="P1 CH1, V" class="DigNum (strict)"("DisabledEnum"=T3."Enabled" ("Disabled")) -> ()  [unwired: 2 in, 2 out]
        n197 = property on="P1 CH1_curlim, A" class="DigNum (strict)"("DisabledEnum"=T3."Enabled" ("Disabled")) -> ()  [unwired: 2 in, 2 out]
        n198 = property on="P1CH1_cur, A" class="DigNum (strict)"("DisabledEnum"=T3."Enabled" ("Disabled")) -> ()  [unwired: 2 in, 2 out]
        n199 = property on="P1 CH1_selcur, A" class="DigNum (strict)"("DisabledEnum"=T3."Enabled" ("Disabled")) -> ()  [unwired: 2 in, 2 out]
        n200 = property on="P1 CH1_counter" class="DigNum (strict)"("DisabledEnum"=T3."Enabled" ("Disabled")) -> ()  [unwired: 2 in, 2 out]
        n201 = property on="P1 CH1_warning" class="Bool (strict)"("DisabledEnum"=T3."Enabled" ("Disabled")) -> ()  [unwired: 2 in, 2 out]
      }
    }
    n202 = local read "STOP"() -> (w270:bool)
    n203 = local read "STOP"() -> (w267:bool)
    n204 = Or(x="P2 CH0 Used", y=w267) -> (x .or. y?=w269:bool)
    n205 = Or(x="P2 CH1 Used", y=w270) -> (x .or. y?=w271:bool)
    n206 = case shown="True" w269 {
      frame False {
        n207 = property on="P2 CH0" class="Bool (strict)"("DisabledEnum"=T3."Disabled and Grayed Out" ("Disabled")) -> ()  [unwired: 2 in, 2 out]
        n208 = property on="P2 CH0_char" class="WFChart (strict)"("DisabledEnum"=T3."Disabled and Grayed Out" ("Disabled")) -> ()  [unwired: 2 in, 2 out]
        n209 = property on="P2 CH0, V" class="DigNum (strict)"("DisabledEnum"=T3."Disabled and Grayed Out" ("Disabled")) -> ()  [unwired: 2 in, 2 out]
        n210 = property on="P2 CH0_curlim, A" class="DigNum (strict)"("DisabledEnum"=T3."Disabled and Grayed Out" ("Disabled")) -> ()  [unwired: 2 in, 2 out]
        n211 = property on="P2 CH0_cur, A" class="DigNum (strict)"("DisabledEnum"=T3."Disabled and Grayed Out" ("Disabled")) -> ()  [unwired: 2 in, 2 out]
        n212 = property on="P2 CH0_selcur, A" class="DigNum (strict)"("DisabledEnum"=T3."Disabled and Grayed Out" ("Disabled")) -> ()  [unwired: 2 in, 2 out]
        n213 = property on="P2 CH0_counter" class="DigNum (strict)"("DisabledEnum"=T3."Disabled and Grayed Out" ("Disabled")) -> ()  [unwired: 2 in, 2 out]
        n214 = property on="P2 CH0_warning" class="Bool (strict)"("DisabledEnum"=T3."Disabled and Grayed Out" ("Disabled")) -> ()  [unwired: 2 in, 2 out]
      }
      frame True {
        n215 = property on="P2 CH0" class="Bool (strict)"("DisabledEnum"=T3."Enabled" ("Disabled")) -> ()  [unwired: 2 in, 2 out]
        n216 = property on="P2 CH0_char" class="WFChart (strict)"("DisabledEnum"=T3."Enabled" ("Disabled")) -> ()  [unwired: 2 in, 2 out]
        n217 = property on="P2 CH0, V" class="DigNum (strict)"("DisabledEnum"=T3."Enabled" ("Disabled")) -> ()  [unwired: 2 in, 2 out]
        n218 = property on="P2 CH0_curlim, A" class="DigNum (strict)"("DisabledEnum"=T3."Enabled" ("Disabled")) -> ()  [unwired: 2 in, 2 out]
        n219 = property on="P2 CH0_cur, A" class="DigNum (strict)"("DisabledEnum"=T3."Enabled" ("Disabled")) -> ()  [unwired: 2 in, 2 out]
        n220 = property on="P2 CH0_selcur, A" class="DigNum (strict)"("DisabledEnum"=T3."Enabled" ("Disabled")) -> ()  [unwired: 2 in, 2 out]
        n221 = property on="P2 CH0_counter" class="DigNum (strict)"("DisabledEnum"=T3."Enabled" ("Disabled")) -> ()  [unwired: 2 in, 2 out]
        n222 = property on="P2 CH0_warning" class="Bool (strict)"("DisabledEnum"=T3."Enabled" ("Disabled")) -> ()  [unwired: 2 in, 2 out]
      }
    }
    n223 = case shown="True" w271 {
      frame False {
        n224 = property on="P2 CH1" class="Bool (strict)"("DisabledEnum"=T3."Disabled and Grayed Out" ("Disabled")) -> ()  [unwired: 2 in, 2 out]
        n225 = property on="P2 CH1_char" class="WFChart (strict)"("DisabledEnum"=T3."Disabled and Grayed Out" ("Disabled")) -> ()  [unwired: 2 in, 2 out]
        n226 = property on="P2 CH1, V" class="DigNum (strict)"("DisabledEnum"=T3."Disabled and Grayed Out" ("Disabled")) -> ()  [unwired: 2 in, 2 out]
        n227 = property on="P2 CH1_curlim, A" class="DigNum (strict)"("DisabledEnum"=T3."Disabled and Grayed Out" ("Disabled")) -> ()  [unwired: 2 in, 2 out]
        n228 = property on="P2 CH1_cur, A" class="DigNum (strict)"("DisabledEnum"=T3."Disabled and Grayed Out" ("Disabled")) -> ()  [unwired: 2 in, 2 out]
        n229 = property on="P2 CH1_selcur, A" class="DigNum (strict)"("DisabledEnum"=T3."Disabled and Grayed Out" ("Disabled")) -> ()  [unwired: 2 in, 2 out]
        n230 = property on="P2 CH1_counter" class="DigNum (strict)"("DisabledEnum"=T3."Disabled and Grayed Out" ("Disabled")) -> ()  [unwired: 2 in, 2 out]
        n231 = property on="P2 CH1_warning" class="Bool (strict)"("DisabledEnum"=T3."Disabled and Grayed Out" ("Disabled")) -> ()  [unwired: 2 in, 2 out]
      }
      frame True {
        n232 = property on="P2 CH1" class="Bool (strict)"("DisabledEnum"=T3."Enabled" ("Disabled")) -> ()  [unwired: 2 in, 2 out]
        n233 = property on="P2 CH1_char" class="WFChart (strict)"("DisabledEnum"=T3."Enabled" ("Disabled")) -> ()  [unwired: 2 in, 2 out]
        n234 = property on="P2 CH1, V" class="DigNum (strict)"("DisabledEnum"=T3."Enabled" ("Disabled")) -> ()  [unwired: 2 in, 2 out]
        n235 = property on="P2 CH1_curlim, A" class="DigNum (strict)"("DisabledEnum"=T3."Enabled" ("Disabled")) -> ()  [unwired: 2 in, 2 out]
        n236 = property on="P2 CH1_cur, A" class="DigNum (strict)"("DisabledEnum"=T3."Enabled" ("Disabled")) -> ()  [unwired: 2 in, 2 out]
        n237 = property on="P2 CH1_selcur, A" class="DigNum (strict)"("DisabledEnum"=T3."Enabled" ("Disabled")) -> ()  [unwired: 2 in, 2 out]
        n238 = property on="P2 CH1_counter" class="DigNum (strict)"("DisabledEnum"=T3."Enabled" ("Disabled")) -> ()  [unwired: 2 in, 2 out]
        n239 = property on="P2 CH1_warning" class="Bool (strict)"("DisabledEnum"=T3."Enabled" ("Disabled")) -> ()  [unwired: 2 in, 2 out]
      }
    }
    n240 = local read "STOP"() -> (w274:bool)
  }
  n241 = while {
    shift-right: [w350] -> _
    shift-left: FALSE -> [w356]
    tunnel: w19 -> [_]
    tunnel: w18 -> [_]
    shift-right: [w349] -> _
    shift-left: FALSE -> [w355]
    shift-right: [w351] -> _
    shift-left: FALSE -> [w354]
    shift-right: [w352] -> _
    shift-left: FALSE -> [w353]
    tunnel: w6 -> [_]
    tunnel: w5 -> [_]
    tunnel: w11 -> [_]
    shift-right: [w345] -> _
    shift-left: FALSE -> [w346]
    shift-right: [w343] -> _
    shift-left: FALSE -> [w344]
    shift-right: [w341] -> _
    shift-left: FALSE -> [w342]
    shift-right: [w339] -> _
    shift-left: FALSE -> [w340]
    stop <- w347 stop-if-true
    # "Включение / выключение образцов"
    n242 = stacked-sequence {
      tunnel: w356 -> [w400 _]
      tunnel: [w396 _] -> w350
      tunnel: w355 -> [w392 _]
      tunnel: [w391 _] -> w349
      tunnel: w354 -> [w390 _]
      tunnel: w353 -> [w384 _]
      tunnel: [w382 _] -> w352
      tunnel: [w381 _] -> w351
      tunnel: [_ w417] -> w347
      tunnel: w346 -> [w378 _]
      tunnel: [w375 _] -> w345
      tunnel: w344 -> [w374 _]
      tunnel: [w369 _] -> w343
      tunnel: w342 -> [w364 _]
      tunnel: [w363 _] -> w341
      tunnel: w340 -> [w358 _]
      tunnel: [w359 _] -> w339
      frame #0 {
        n243 = local read "P1 CH0 Used"() -> (w375:bool)
        n244 = local read "P1 CH1 Used"() -> (w369:bool)
        n245 = local read "P2 CH0 Used"() -> (w363:bool)
        n246 = local read "P2 CH1 Used"() -> (w359:bool)
        n247 = local read "P1 CH1"() -> (w381:bool)
        n248 = local read "P2 CH1"() -> (w396:bool)
        n249 = local read "P2 CH0"() -> (w391:bool)
        n250 = local read "P1 CH0"() -> (w382:bool)
        n251 = local read "STOP"() -> (w371:bool)
        n252 = local read "STOP"() -> (w366:bool)
        n253 = local read "STOP"() -> (w379:bool)
        n254 = Less?(x=w381, y=w390) -> (x < y?=w372:bool)
        n255 = Less?(x=w396, y=w400) -> (x < y?=w362:bool)
        n256 = Less?(x=w391, y=w392) -> (x < y?=w368:bool)
        n257 = Less?(x=w363, y=w364) -> (x < y?=w365:bool)
        n258 = Less?(x=w382, y=w384) -> (x < y?=w380:bool)
        n259 = Not(x=w371) -> (.not. x?=w389:bool)
        n260 = Greater?(x=w381, y=w390) -> (0:w388:bool)
        n261 = Not(x="STOP") -> (.not. x?=w398:bool)
        n262 = Not(x=w366) -> (.not. x?=w394:bool)
        n263 = Greater?(x=w396, y=w400) -> (0:w397:bool)
        n264 = Not(x=w379) -> (.not. x?=w385:bool)
        n265 = Greater?(x=w391, y=w392) -> (0:w395:bool)
        n266 = Greater?(x=w382, y=w384) -> (0:w386:bool)
        n267 = Less?(x=w359, y=w358) -> (x < y?=w357:bool)
        n268 = Less?(x=w375, y=w378) -> (x < y?=w377:bool)
        n269 = Less?(x=w369, y=w374) -> (x < y?=w370:bool)
        n270 = And(x=w389, y=w388) -> (x .and. y?=w387:bool)
        n271 = Compound Arithmetic op=OR(w368, w366, w365) -> (w367:bool)
        n272 = And(x=w398, y=w397) -> (x .and. y?=w399:bool)
        n273 = And(x=w394, y=w395) -> (x .and. y?=w393:bool)
        n274 = Compound Arithmetic op=OR(w362, "STOP", w357) -> (w360:bool)
        n275 = And(x=w385, y=w386) -> (x .and. y?=w383:bool)
        n276 = Compound Arithmetic op=OR(w380, w379, w377) -> (w376:bool)
        n277 = Compound Arithmetic op=OR(w372, w371, w370) -> (w373:bool)
        n278 = stacked-sequence {
          tunnel: w383 -> [w406]
          tunnel: w376 -> [w405]
          frame #0 {
            n279 = case shown="True" w406 {
              frame False {
              }
              frame True {
                # "ON"
                n280 = local write "P1 CH0"(TRUE ("P1 CH0")) -> ()
              }
            }
            n281 = case shown="True" w405 {
              frame False {
              }
              frame True {
                # "OFF"
                n282 = local write "P1 CH0"(FALSE ("P1 CH0")) -> ()
              }
            }
          }
        }
        n283 = stacked-sequence {
          tunnel: w387 -> [w402]
          tunnel: w373 -> [w401]
          frame #0 {
            n284 = case shown="True" w402 {
              frame False {
              }
              frame True {
                # "ON"
                n285 = local write "P1 CH1"(TRUE ("P1 CH1")) -> ()
              }
            }
            n286 = case shown="True" w401 {
              frame False {
              }
              frame True {
                # "OFF"
                n287 = local write "P1 CH1"(FALSE ("P1 CH0")) -> ()
              }
            }
          }
        }
        n288 = stacked-sequence {
          tunnel: w393 -> [w410]
          tunnel: w367 -> [w409]
          frame #0 {
            n289 = case shown="True" w410 {
              frame False {
              }
              frame True {
                # "ON"
                n290 = local write "P2 CH0"(TRUE ("P2 CH0")) -> ()
              }
            }
            n291 = case shown="True" w409 {
              frame False {
              }
              frame True {
                # "OFF"
                n292 = local write "P2 CH0"(FALSE ("P1 CH0")) -> ()
              }
            }
          }
        }
        n293 = stacked-sequence {
          tunnel: w399 -> [w414]
          tunnel: w360 -> [w413]
          frame #0 {
            n294 = case shown="True" w414 {
              frame False {
              }
              frame True {
                # "ON"
                n295 = local write "P2 CH1"(TRUE ("P2 CH1")) -> ()
              }
            }
            n296 = case shown="True" w413 {
              frame False {
              }
              frame True {
                # "OFF"
                n297 = local write "P2 CH1"(FALSE ("P1 CH0")) -> ()
              }
            }
          }
        }
      }
      frame #1 {
        n298 = local read "STOP"() -> (w417:bool)
      }
    }
    "Power OFF" <- w347
    n299 = Wait (ms)(milliseconds to wait=u32 1) -> ()  [unwired: 1 out]
  }
  n300 = while {
    shift-right: [w425] -> _
    shift-left: FALSE -> [w429]
    tunnel: w6 -> [w428]
    tunnel: [w427] -> _
    tunnel: [w426] -> w9
    tunnel: w19 -> [_]
    tunnel: w18 -> [_]
    shift-right: [w423] -> _
    shift-left: FALSE -> [w424]
    shift-right: [w421] -> _
    shift-left: FALSE -> [w422]
    shift-right: [w420] -> _
    shift-left: FALSE -> [w419]
    tunnel: w5 -> [_]
    tunnel: w11 -> [_]
    stop <- w427 stop-if-true
    n301 = Wait (ms)(milliseconds to wait="SEL Time Cycle") -> ()  [unwired: 1 out]
    n302 = stacked-sequence {
      seq-local: [w433 _ _ _] -> [_ _ w598 _]
      seq-local: [w432 _ _ _] -> [_ _ w595 _]
      seq-local: [w431 _ _ _] -> [_ _ w593 _]
      seq-local: [w430 _ _ _] -> [_ _ w592 _]
      tunnel: w429 -> [w441 _ _ _]
      tunnel: [_ _ _ w625] -> w427
      tunnel: w428 -> [_ w581 _ _]
      tunnel: [_ w580 _ _] -> w426
      tunnel: [_ _ w600 _] -> w425
      tunnel: w424 -> [w439 _ _ _]
      tunnel: [_ _ w594 _] -> w423
      tunnel: w422 -> [w438 _ _ _]
      tunnel: [_ _ w596 _] -> w421
      tunnel: [_ _ w597 _] -> w420
      tunnel: w419 -> [w434 _ _ _]
      frame #0 {
        # "Детектирование SEL"
        n303 = local read "P2 CH0"() -> (w432:bool)
        n304 = local read "P1 CH1"() -> (w431:bool)
        n305 = local read "P2 CH1"() -> (w433:bool)
        n306 = flat-sequence {
          tunnel: w436 -> [w474]
          frame #0 {
            n307 = case shown="True" w474 {
              frame False {
              }
              frame True {
                n308 = Wait (ms)(milliseconds to wait=u32 50) -> ()  [unwired: 1 out]
              }
            }
          }
          frame #1 {
            n309 = local read "P1CH1_cur, A"() -> (w479:dbl)
            n310 = local read "SIM_SEL"() -> (w477:bool)
            n311 = Greater Or Equal?(x=w479, y="P1 CH1_selcur, A") -> (x >= y?=w480:bool)
            n312 = Or(x=w477, y=w480) -> (x .or. y?=→"P1 CH1_warning":bool)
          }
          frame #2 {
            n313 = local read "Считать SIM_SEL"() -> (w486:bool)
            n314 = local read "SIM_SEL"() -> (w485:bool)
            n315 = local read "P1 CH1_warning"() -> (w481:bool)
            n316 = Not(x=w485) -> (.not. x?=w484:bool)
            n317 = Select(t=TRUE, s=w486, f=w484) -> (s? t:f=w482:bool)
            n318 = And(x=w481, y=w482) -> (x .and. y?=w487:bool)
            n319 = case shown="True" w487 {
              frame False {
              }
              frame True {
                n320 = local read "P1 CH1_counter"() -> (w489:u32)
                n321 = Increment(x=w489) -> (x+1=→"P1 CH1_counter":u32)
              }
            }
          }
        }
        n322 = flat-sequence {
          tunnel: w437 -> [w458]
          frame #0 {
            n323 = case shown="True" w458 {
              frame False {
              }
              frame True {
                n324 = Wait (ms)(milliseconds to wait=u32 50) -> ()  [unwired: 1 out]
              }
            }
          }
          frame #1 {
            n325 = local read "P2 CH0_cur, A"() -> (w464:dbl)
            n326 = local read "SIM_SEL"() -> (w461:bool)
            n327 = Greater Or Equal?(x=w464, y="P2 CH0_selcur, A") -> (x >= y?=w463:bool)
            n328 = Or(x=w461, y=w463) -> (x .or. y?=→"P2 CH0_warning":bool)
          }
          frame #2 {
            n329 = local read "Считать SIM_SEL"() -> (w468:bool)
            n330 = local read "SIM_SEL"() -> (w469:bool)
            n331 = local read "P2 CH0_warning"() -> (w465:bool)
            n332 = Not(x=w469) -> (.not. x?=w470:bool)
            n333 = Select(t=TRUE, s=w468, f=w470) -> (s? t:f=w467:bool)
            n334 = And(x=w465, y=w467) -> (x .and. y?=w466:bool)
            n335 = case shown="True" w466 {
              frame False {
              }
              frame True {
                n336 = local read "P2 CH0_counter"() -> (w473:u32)
                n337 = Increment(x=w473) -> (x+1=→"P2 CH0_counter":u32)
              }
            }
          }
        }
        n338 = flat-sequence {
          tunnel: w440 -> [w490]
          frame #0 {
            n339 = case shown="True" w490 {
              frame False {
              }
              frame True {
                n340 = Wait (ms)(milliseconds to wait=u32 50) -> ()  [unwired: 1 out]
              }
            }
          }
          frame #1 {
            n341 = local read "P1 CH0_cur, A"() -> (w496:dbl)
            n342 = Greater Or Equal?(x=w496, y="P1 CH0_selcur, A") -> (x >= y?=w495:bool)
            n343 = Or(x="SIM_SEL", y=w495) -> (x .or. y?=→"P1 CH0_warning":bool)
          }
          frame #2 {
            n344 = local read "SIM_SEL"() -> (w502:bool)
            n345 = local read "P1 CH0_warning"() -> (w497:bool)
            n346 = Not(x=w502) -> (.not. x?=w501:bool)
            n347 = Select(t=TRUE, s="Считать SIM_SEL", f=w501) -> (s? t:f=w498:bool)
            n348 = And(x=w497, y=w498) -> (x .and. y?=w503:bool)
            n349 = case shown="True" w503 {
              frame False {
              }
              frame True {
                n350 = local read "P1 CH0_counter"() -> (w505:u32)
                n351 = Increment(x=w505) -> (x+1=→"P1 CH0_counter":u32)
              }
            }
          }
        }
        n352 = flat-sequence {
          tunnel: w435 -> [w442]
          frame #0 {
            n353 = case shown="True" w442 {
              frame False {
              }
              frame True {
                n354 = Wait (ms)(milliseconds to wait=u32 50) -> ()  [unwired: 1 out]
              }
            }
          }
          frame #1 {
            n355 = local read "P2 CH1_cur, A"() -> (w446:dbl)
            n356 = local read "SIM_SEL"() -> (w444:bool)
            n357 = Greater Or Equal?(x=w446, y="P2 CH1_selcur, A") -> (x >= y?=w447:bool)
            n358 = Or(x=w444, y=w447) -> (x .or. y?=→"P2 CH1_warning":bool)
          }
          frame #2 {
            n359 = local read "Считать SIM_SEL"() -> (w455:bool)
            n360 = local read "SIM_SEL"() -> (w454:bool)
            n361 = local read "P2 CH1_warning"() -> (w449:bool)
            n362 = Not(x=w454) -> (.not. x?=w453:bool)
            n363 = Select(t=TRUE, s=w455, f=w453) -> (s? t:f=w451:bool)
            n364 = And(x=w449, y=w451) -> (x .and. y?=w450:bool)
            n365 = case shown="True" w450 {
              frame False {
              }
              frame True {
                n366 = local read "P2 CH1_counter"() -> (w457:u32)
                n367 = Increment(x=w457) -> (x+1=→"P2 CH1_counter":u32)
              }
            }
          }
        }
        n368 = local read "P1 CH0"() -> (w430:bool)
        n369 = Greater?(x=w432, y=w438) -> (0:w437:bool)
        n370 = Greater?(x=w430, y=w441) -> (0:w440:bool)
        n371 = Greater?(x=w431, y=w439) -> (0:w436:bool)
        n372 = Greater?(x=w433, y=w434) -> (0:w435:bool)
      }
      frame #1 {
        w507 = "\t"
        w519 = "\t"
        w521 = "\t"
        w523 = "\t"
        w508 = "\t"
        w509 = "\t"
        w510 = "\t"
        w511 = "\t"
        w554 = 0
        w553 = 6
        w549 = 6
        w559 = 0
        w560 = 6
        w564 = 6
        w573 = 0
        w572 = 6
        w567 = 6
        w576 = 0
        w577 = 6
        w584 = 6
        # "Запись логов"
        n373 = local read "P2 CH1, V"() -> (w556:dbl)
        n374 = local read "P2 CH1_cur, A"() -> (w552:dbl)
        n375 = local read "P2 CH1_counter"() -> (w555:u32)
        n376 = local read "P2 CH1_warning"() -> (w551:bool)
        n377 = local read "P1 CH0, V"() -> (w582:dbl)
        n378 = local read "P1 CH0_cur, A"() -> (w578:dbl)
        n379 = local read "P1 CH0_counter"() -> (w575:u32)
        n380 = local read "P1 CH0_warning"() -> (w579:bool)
        n381 = local read "P1 CH1, V"() -> (w569:dbl)
        n382 = local read "P1CH1_cur, A"() -> (w571:dbl)
        n383 = local read "P1 CH1_counter"() -> (w574:u32)
        n384 = local read "P1 CH1_warning"() -> (w570:bool)
        n385 = local read "P2 CH0, V"() -> (w557:dbl)
        n386 = local read "P2 CH0_cur, A"() -> (w561:dbl)
        n387 = local read "P2 CH0_counter"() -> (w558:u32)
        n388 = local read "P2 CH0_warning"() -> (w562:bool)
        n389 = Number To Fractional String(number=w556, width (-)=w549, precision (6)=w549) -> (F-format string=w535:string)  [unwired: 1 in]
        n390 = Number To Fractional String(number=w552, width (-)=w553, precision (6)=w553) -> (F-format string=w534:string)  [unwired: 1 in]
        n391 = Number To Fractional String(number=w555, width (-)=w554, precision (6)=w554) -> (F-format string=w533:string)  [unwired: 1 in]
        n392 = Number To Fractional String(number=w582, width (-)=w584, precision (6)=w584) -> (F-format string=w547:string)  [unwired: 1 in]
        n393 = Number To Fractional String(number=w578, width (-)=w577, precision (6)=w577) -> (F-format string=w546:string)  [unwired: 1 in]
        n394 = Number To Fractional String(number=w575, width (-)=w576, precision (6)=w576) -> (F-format string=w545:string)  [unwired: 1 in]
        n395 = Number To Fractional String(number=w569, width (-)=w567, precision (6)=w567) -> (F-format string=w543:string)  [unwired: 1 in]
        n396 = Number To Fractional String(number=w571, width (-)=w572, precision (6)=w572) -> (F-format string=w542:string)  [unwired: 1 in]
        n397 = Number To Fractional String(number=w574, width (-)=w573, precision (6)=w573) -> (F-format string=w541:string)  [unwired: 1 in]
        n398 = Number To Fractional String(number=w557, width (-)=w564, precision (6)=w564) -> (F-format string=w539:string)  [unwired: 1 in]
        n399 = Number To Fractional String(number=w561, width (-)=w560, precision (6)=w560) -> (F-format string=w538:string)  [unwired: 1 in]
        n400 = Number To Fractional String(number=w558, width (-)=w559, precision (6)=w559) -> (F-format string=w537:string)  [unwired: 1 in]
        n401 = Select(t="!!!3", s=w551, f="") -> (s? t:f=w532:string)
        n402 = Select(t="!!!0", s=w579, f="") -> (s? t:f=w544:string)
        n403 = Select(t="!!!1", s=w570, f="") -> (s? t:f=w540:string)
        n404 = Select(t="!!!2", s=w562, f="") -> (s? t:f=w536:string)
        n405 = local read "P1 CH0 Used"() -> (w528:bool)
        n406 = local read "P1 CH1 Used"() -> (w527:bool)
        n407 = local read "P2 CH0 Used"() -> (w526:bool)
        n408 = local read "P2 CH1 Used"() -> (w525:bool)
        n409 = Concatenate Strings(w511, w547, w511, w546, w511, w545, w511, w544) -> (w530:string)
        n410 = Concatenate Strings(w510, w543, w510, w542, w510, w541, w510, w540) -> (w531:string)
        n411 = Concatenate Strings(w509, w539, w509, w538, w509, w537, w509, w536) -> (w529:string)
        n412 = Concatenate Strings(w508, w535, w508, w534, w508, w533, w508, w532) -> (w524:string)
        n413 = Concatenate Strings(w523, w523, w523, w523) -> (w522:string)
        n414 = Concatenate Strings(w521, w521, w521, w521) -> (w520:string)
        n415 = Concatenate Strings(w519, w519, w519, w519) -> (w518:string)
        n416 = Concatenate Strings(w507, w507, w507, w507) -> (w517:string)
        n417 = Select(t=w530, s=w528, f=w522) -> (s? t:f=w516:string)
        n418 = Select(t=w531, s=w527, f=w520) -> (s? t:f=w515:string)
        n419 = Select(t=w529, s=w526, f=w518) -> (s? t:f=w514:string)
        n420 = Select(t=w524, s=w525, f=w517) -> (s? t:f=w513:string)
        n421 = Get Date/Time In Seconds() -> (seconds since 1Jan1904=w587:timestamp)
        n422 = Format Date/Time String(time format string (%c)="%H:%M:%S:%3u", seconds (now)=w587) -> (date/time string=w585:string)  [unwired: 1 in]
        n423 = Concatenate Strings(w585, w516, w515, w514, w513, "\r\n") -> (w512:string)
        n424 = Format Into String(initial string=w581, w512) -> (resulting string=w580:refnum<file>)  [unwired: 2 in, 1 out]
      }
      frame #2 {
        n425 = local read "P1 CH0_warning"() -> (w599:bool)
        "SEL" <- w599
        n426 = local read "P1 CH1_warning"() -> (w591:bool)
        n427 = local read "P2 CH0_warning"() -> (w589:bool)
        n428 = local read "P2 CH1_warning"() -> (w590:bool)
        n429 = local write "SEL"(w589) -> ()
        n430 = local write "SEL"(w591) -> ()
        n431 = local write "SEL"(w590) -> ()
        n432 = case shown="True" w599 {
          tunnel: [w619 w620] -> w600
          tunnel: w592 -> [w619 _]
          frame False {
          }
          frame True {
            n433 = flat-sequence {
              tunnel: [FALSE] -> w620
              frame #0 {
                n434 = local write "P1 CH0"(FALSE ("Power")) -> ()
              }
              frame #1 {
                n435 = Wait (ms)(milliseconds to wait=u32 100 ("Wait_parry, ms")) -> ()  [unwired: 1 out]
              }
              frame #2 {
                n436 = local write "P1 CH0"(TRUE ("Power")) -> ()
              }
            }
          }
        }
        n437 = case shown="True" w591 {
          tunnel: [w613 w614] -> w594
          tunnel: w593 -> [w613 _]
          frame False {
          }
          frame True {
            n438 = flat-sequence {
              tunnel: [FALSE] -> w614
              frame #0 {
                n439 = local write "P1 CH1"(FALSE ("Power")) -> ()
              }
              frame #1 {
                n440 = Wait (ms)(milliseconds to wait=u32 100 ("Wait_parry, ms")) -> ()  [unwired: 1 out]
              }
              frame #2 {
                n441 = local write "P1 CH1"(TRUE ("Power")) -> ()
              }
            }
          }
        }
        n442 = case shown="True" w589 {
          tunnel: [w607 w608] -> w596
          tunnel: w595 -> [w607 _]
          frame False {
          }
          frame True {
            n443 = flat-sequence {
              tunnel: [FALSE] -> w608
              frame #0 {
                n444 = local write "P2 CH0"(FALSE ("Power")) -> ()
              }
              frame #1 {
                n445 = Wait (ms)(milliseconds to wait=u32 100 ("Wait_parry, ms")) -> ()  [unwired: 1 out]
              }
              frame #2 {
                n446 = local write "P2 CH0"(TRUE ("Power")) -> ()
              }
            }
          }
        }
        n447 = case shown="True" w590 {
          tunnel: [w601 w602] -> w597
          tunnel: w598 -> [w601 _]
          frame False {
          }
          frame True {
            n448 = flat-sequence {
              tunnel: [FALSE] -> w602
              frame #0 {
                n449 = local write "P2 CH1"(FALSE ("Power")) -> ()
              }
              frame #1 {
                n450 = Wait (ms)(milliseconds to wait=u32 100 ("Wait_parry, ms")) -> ()  [unwired: 1 out]
              }
              frame #2 {
                n451 = local write "P2 CH1"(TRUE ("Power")) -> ()
              }
            }
          }
        }
      }
      frame #3 {
        n452 = local read "STOP"() -> (w625:bool)
      }
    }
  }
  n453 = while {
    tunnel: w11 -> [w639]
    tunnel: [w644] -> w7
    tunnel: w5 -> [w634]
    tunnel: [w632] -> w8
    tunnel: w6 -> [_]
    stop <- w640 stop-if-true
    n454 = flat-sequence {
      tunnel: w639 -> [w649]
      tunnel: [w645] -> w627
      tunnel: [w654] -> w643
      tunnel: w627 -> [w653]
      tunnel: [w661] -> w642
      tunnel: w643 -> [w660]
      tunnel: w642 -> [w663]
      tunnel: [w662] -> w641
      tunnel: [w678] -> w637
      tunnel: w641 -> [w680]
      tunnel: [w677] -> w635
      tunnel: [w670] -> w630
      tunnel: [w672] -> w629
      tunnel: [w671] -> w628
      tunnel: [w667] -> w626
      tunnel: w637 -> [w737]
      tunnel: [w737] -> w636
      tunnel: w635 -> [w719]
      tunnel: w634 -> [w727]
      tunnel: [w726] -> w633
      tunnel: [w724] -> w631
      tunnel: w630 -> [w723]
      tunnel: w629 -> [w722]
      tunnel: w628 -> [w721]
      tunnel: w626 -> [w717]
      tunnel: [w742] -> w644
      tunnel: w636 -> [w742]
      tunnel: [w743] -> w640
      tunnel: w633 -> [w741]
      tunnel: [w741] -> w632
      tunnel: w631 -> [_]
      frame #0 {
        n455 = call <instrlib>:"niScope Configure Vertical.vi"("instrument handle"=w649, "probe attenuation"=1.0 ("Probe Attenuation"), "vertical coupling"="AC/DC/Groun", "channels"="0" ("Channel Name"), "vertical offset"=0.0 ("Vertical Offset")) -> ("instrument handle out"=w645:refnum<k15>)  [unwired: 9 in, 1 out]
      }
      frame #1 {
        w659 = 0 items=["Positive", "Negative"] ("Trigger Slope")
        w658 = u16 1 items=["AC"=0, "DC"=1, "HF Reject"=3, "LF Reject"=4, "AC Plus HF Reject"=1001] ("Coupling")
        n456 = call-poly <instrlib>:"niScope Configure Trigger (poly).vi"("instrument handle"=w653, "trigger window mode"=w659, "trigger coupling"=w658, "trigger source"="Trigger Source", "low level"="Low Level", "high level"="High Level", "trigger holdoff"=0.0, "trigger delay"=0.0 ("Trigger Delay")) -> ("instrument handle out"=w654:refnum<k15>)  [unwired: 6 in, 1 out]
      }
      frame #2 {
        n457 = call <instrlib>:"niScope Initiate Acquisition.vi"("instrument handle"=w660) -> ("instrument handle out"=w661:refnum<k15>)  [unwired: 13 in, 1 out]
      }
      frame #3 {
        n458 = call-poly <instrlib>:"niScope Fetch (poly).vi"("timeout"=1.0, "channels"="0", "instrument handle"=w663) -> ("waveform"=→"RealTime Waveform":T2, "instrument handle out"=w662:refnum<k15>)  [unwired: 5 in, 2 out]
      }
      frame #4 {
        # "Во время триггера FALSE"
        n459 = property class="niScope"(reference=w680) -> (reference out=w679:refnum<k15>, "Auto Triggered"=w676:bool)  [unwired: 1 in, 1 out]
        n460 = case shown="\"Radio Selection P1 CH0\", Default" "Channel for SEU" {
          tunnel: [w682 w688 w690 w694] -> w672
          tunnel: [w683 w687 w691 w695] -> w671
          tunnel: [w684 w686 w692 w696] -> w670
          tunnel: [w681 w685 w689 w693] -> w668
          frame "Radio Selection P1 CH0", Default {
            n461 = local read "P1 CH0_warning"() -> (w681:bool)
            n462 = local read "P1 CH0_cur, A"() -> (w682:dbl)
            n463 = local read "P1 CH0, V"() -> (w683:dbl)
            n464 = Get Date/Time In Seconds() -> (seconds since 1Jan1904=w684:timestamp)
          }
          frame "Radio Selection P1 CH1" {
            n465 = local read "P1 CH1_warning"() -> (w685:bool)
            n466 = local read "P1CH1_cur, A"() -> (w688:dbl)
            n467 = local read "P1 CH1, V"() -> (w687:dbl)
            n468 = Get Date/Time In Seconds() -> (seconds since 1Jan1904=w686:timestamp)
          }
          frame "Radio Selection P2 CH0" {
            n469 = local read "P2 CH0_warning"() -> (w689:bool)
            n470 = local read "P2 CH0_cur, A"() -> (w690:dbl)
            n471 = local read "P2 CH0, V"() -> (w691:dbl)
            n472 = Get Date/Time In Seconds() -> (seconds since 1Jan1904=w692:timestamp)
          }
          frame "Radio Selection P2 CH1" {
            n473 = local read "P1 CH1_warning"() -> (w693:bool)
            n474 = local read "P2 CH1_cur, A"() -> (w694:dbl)
            n475 = local read "P2 CH1, V"() -> (w695:dbl)
            n476 = Get Date/Time In Seconds() -> (seconds since 1Jan1904=w696:timestamp)
          }
        }
        n477 = Not(x=w676) -> (.not. x?=w675:bool)
        n478 = Not(x=w668) -> (.not. x?=w673:bool)
        n479 = And(x=w673, y=w675) -> (x .and. y?=w674:bool)
        n480 = case shown="True" w674 {
          tunnel: w679 -> [w699 w711]
          tunnel: [w699 w703] -> w678
          tunnel: [FALSE TRUE] -> w677
          tunnel: ["" w700] -> w667
          frame False {
          }
          frame True {
            w702 = 6
            # "Регистрация SEU"
            n481 = call-poly <instrlib>:"niScope Fetch (poly).vi"("timeout"=1.0, "channels"="0", "instrument handle"=w711) -> ("waveform"=→"SEU Waveform":T2, "instrument handle out"=w704:refnum<k15>)  [unwired: 5 in, 2 out]
            n482 = call-poly <instrlib>:"niScope Fetch (poly).vi"("timeout"=1.0, "numSamples"=1, "channels"="0", "instrument handle"=w704) -> ("wfm"=w709:dbl[], "instrument handle out"=w703:refnum<k15>)  [unwired: 4 in, 2 out]
            n483 = Index Array(array=w709, index=0) -> (element=w701:dbl)
            "SEU last level" <- w701
            n484 = Number To Fractional String(number=w701, width (-)=w702, precision (6)=w702) -> (F-format string=w700:string)  [unwired: 1 in]
          }
        }
      }
      frame #5 {
        w728 = 6
        w732 = 0
        w731 = 6
        w718 = "\t"
        # "Регистрация SEU"
        n485 = case shown="True" w719 {
          tunnel: [w738 w739] -> w720
          frame False {
            n486 = local read "SEU_Counter"() -> (w738:u32)
          }
          frame True {
            n487 = local read "SEU_Counter"() -> (w740:u32)
            n488 = Increment(x=w740) -> (x+1=w739:u32)
            "SEU_Counter" <- w739
          }
        }
        n489 = Format Date/Time String(time format string (%c)="%H:%M:%S:%3u", seconds (now)=w723) -> (date/time string=w734:string)  [unwired: 1 in]
        n490 = Number To Fractional String(number=w721, width (-)=w728, precision (6)=w728) -> (F-format string=w733:string)  [unwired: 1 in]
        n491 = Number To Fractional String(number=w722, width (-)=w731, precision (6)=w731) -> (F-format string=w735:string)  [unwired: 1 in]
        n492 = Number To Fractional String(number=w720, width (-)=w732, precision (6)=w732) -> (F-format string=w736:string)  [unwired: 1 in]
        n493 = Select(t="???", s=w719, f="") -> (s? t:f=w716:string)
        n494 = Concatenate Strings(w734, w718, w733, w718, w735, w718, w736, w718, w717, w718, w716, "\r\n") -> (w724:string)
        n495 = Format Into String(initial string=w727, w724) -> (resulting string=w726:refnum<file>)  [unwired: 2 in, 1 out]
        "SEU_warning" <- w719
        "SEU" <- w719
      }
      frame #6 {
        n496 = local read "STOP"() -> (w743:bool)
      }
    }
    n497 = Wait (ms)(milliseconds to wait=u32 1) -> ()  [unwired: 1 out]
  }
  n498 = flat-sequence {
    tunnel: w9 -> [w746]
    tunnel: w8 -> [w745]
    tunnel: w7 -> [w744]
    frame #0 {
      # "STOP"
      n499 = Close File(refnum=w745) -> ()  [unwired: 1 in, 2 out]
      n500 = Close File(refnum=w746) -> ()  [unwired: 1 in, 2 out]
      n501 = call <instrlib>:"niScope Close.vi"("instrument handle"=w744) -> ()  [unwired: 14 in, 1 out]
      n502 = Wait (ms)(milliseconds to wait=u32 1) -> ()  [unwired: 1 out]
    }
  }
